vi "Invoke folder dialogue 26_01_18.vi"() -> (0 "error out":errorcluster, 3 "Folder exists & not cancelled":bool)   [LabVIEW 2020]
uses:
  Global variables/gl_Functional Imaging-Global variables.vi
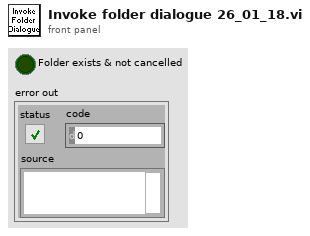
[diagram p1: front panel]
types:
  T1 = typedef "Functional Imging UI Refs.ctl" = cluster{"Menu ref":refnum<k9>, "Image control":refnum<vi>, "VI ref":refnum<vi>, "XGrapher":refnum<vi>, "Smoothing":refnum<vi>, "POI Averaging":refnum<vi>, "Normalize":refnum<vi>, "POI data points in each trial":refnum<vi>, "Channel":refnum<vi>, "Experiment data folder path":refnum<vi>, "[ROI vis]":refnum<vi>, "[Groups] visbl":T2, "Group Name":refnum<vi>, "POI index":refnum<vi>, "Trial No.":refnum<vi>, "Intensity Zoom":refnum<vi>, "Trial Cursor Enabled":refnum<vi>, "Number of Trials (ind 1)":refnum<vi>, "Number of Trials (ind 2)":refnum<vi>, "MiniScans Available":refnum<vi>, "POI Available":refnum<vi>, "Defer graph updates":refnum<vi>, "Waveform selector":refnum<vi>, "#of selected POI":refnum<vi>, "#of selected MiniScans":refnum<vi>, "#of selected groups":refnum<vi>, "Max Z-Projection":refnum<vi>, "Z-Plane Selector":refnum<vi>, "Index of miniscan point to visualise":refnum<vi>, "ROI vis. mode":refnum<vi>, "Total # of points":refnum<vi>, "Index of group clicked on":refnum<vi>, "Pane 1":refnum<vi>, "Pane 2":refnum<vi>, "Pane 3":refnum<vi>, "Pane 4":refnum<vi>, "Pane 5":refnum<vi>, "Pane 6":refnum<vi>, "Deselect all ROI":refnum<vi>, "Deselect all groups":refnum<vi>}
  T2 = typedef "Groups array referecne.ctl" = refnum<vi>
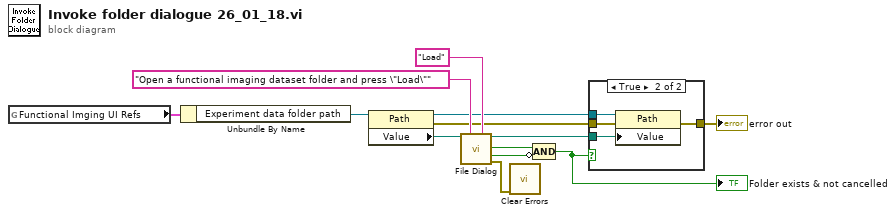
[diagram p0: block diagram]
diagram:
  n1 = global read "gl_Functional Imaging-Global variables.vi" "Functional Imging UI Refs"() -> (w1:T1)
  n2 = Unbundle By Name(w1) -> ("Experiment data folder path"=w9:refnum<vi>)
  n3 = property class="Path"(reference=w9) -> (reference out=w7:refnum<vi>, error out=w2:errorcluster, "Value"=w8:path)  [unwired: 1 in]
  n4 = call "File Dialog"("start path"=w8, "prompt"="Open a functional imaging dataset folder and press \"Load\"", "button label"="Load") -> ("selected path"=w5:path, "exists"=w13:bool, "cancelled"=w12:bool, "error out"=w3:errorcluster)  [unwired: 9 in]
  n5 = call <vilib>:"Clear Errors.vi"("error in (no error)"=w3) -> ()  [unwired: 5 in, 2 out]
  n6 = Compound Arithmetic op=AND(w13, invert w12) -> (w6:bool)
  "Folder exists & not cancelled" <- w6
  n7 = case shown="True" w6 {
    tunnel: w7 -> [_ w18]
    tunnel: w5 -> [_ w17]
    tunnel: [w14 w16] -> w4
    tunnel: w2 -> [w14 w15]
    frame False {
    }
    frame True {
      n8 = property class="Path"(reference=w18, error in=w15, "Value"=w17) -> (error out=w16:errorcluster)  [unwired: 1 out]
    }
  }
  "error out" <- w4
